vi "log appender.vi"(8 "error in (no error)":errorcluster caption="에러 입력(에러 없음)", 11 "GUI Log Class 입력":refnum<class "GUI Log Class.lvclass">) -> (0 "error out":errorcluster caption="에러 출력")   [LabVIEW 2020, in "GUI Log Class.lvclass"]
uses:
  GUI Log Class.lvclass
  GUI Log Class.lvclass/GUI Log Class.ctl
  Controls/line limit fgv enum.ctl
  Accessors/Read log ref.vi
  Accessors/Read appender queue.vi
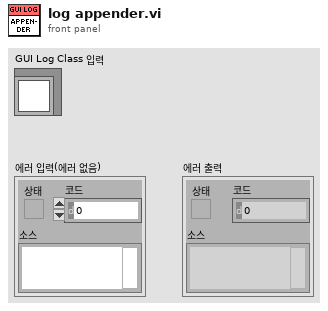
[diagram p1: front panel]
types:
  T1 = typedef "GUI Log Class.lvclass/line limit fgv enum.ctl" = enum16{"Read", "Write"}
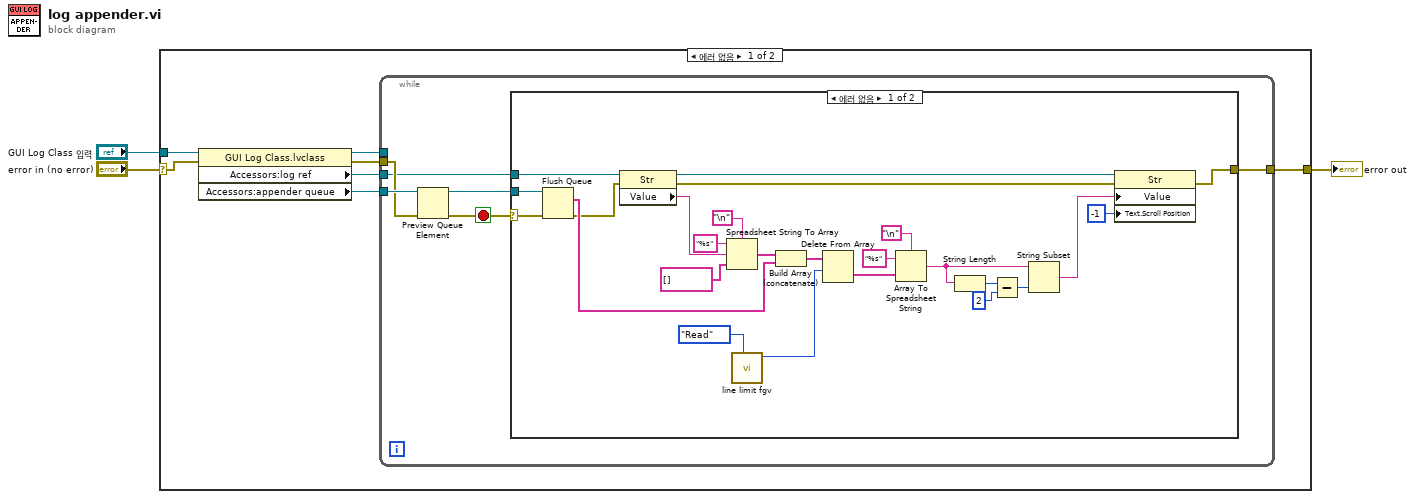
[diagram p0: block diagram]
diagram:
  n1 = case shown="에러 없음" "error in (no error)" {
    selector: "error in (no error)" -> [w10 w43]
    tunnel: [w5 w43] -> w2
    tunnel: "GUI Log Class 입력" -> [w9 _]
    frame No Error {
      n2 = property class="GUI Log Class.lvclass"(reference=w9, error in=w10) -> (reference out=w8:refnum<class "GUI Log Class.lvclass">, error out=w7:errorcluster, "Accessors:log ref"=w4:refnum<vi>, "Accessors:appender queue"=w6:refnum<queue>)
      n3 = while {
        tunnel: w8 -> [_]
        tunnel: w7 -> [w15]
        tunnel: w6 -> [w16]
        tunnel: [w14] -> w5
        tunnel: w4 -> [w11]
        stop <- w12 stop-if-true
        n4 = Preview Queue Element(queue=w16, error in (no error)=w15) -> (queue out=w13:refnum<queue>, error out=w12:errorcluster)  [unwired: 1 in, 2 out]
        n5 = case shown="에러 없음" w12 {
          selector: w12 -> [w40 w42]
          tunnel: [w21 w42] -> w14
          tunnel: w13 -> [w41 _]
          tunnel: w11 -> [w20 _]
          frame No Error {
            n6 = Flush Queue(queue=w41, error in (no error)=w40) -> (remaining elements=w25:string[], error out=w19:errorcluster)  [unwired: 1 out]
            n7 = property class="Str"(reference=w20, error in=w19) -> (reference out=w36:refnum<vi>, error out=w24:errorcluster, "Value"=w31:string)
            n8 = Spreadsheet String To Array(delimiter (Tab)="\n" ("구분 문자 (탭)"), format string="%s" ("포맷 문자열"), spreadsheet string=w31, array type (2D Dbl)=string[] []) -> (array=w27:string[])
            n9 = call "line limit fgv.vi"("function"=line_limit_fgv_enum."Read") -> ("line limit out"=w17:i32)  [unwired: 9 in, 1 out]
            n10 = Build Array (concatenate)(w27, w25) -> (w26:string[])
            n11 = Delete From Array(array=w26, length=w17) -> (deleted portion=w23:string[])  [unwired: 1 in, 1 out]
            n12 = Array To Spreadsheet String(delimiter (Tab)="\n", array=w23, 3:"%s" ("포맷 문자열")) -> (spreadsheet string=w35:string)
            n13 = String Length(string=w35) -> (length=w34:i32)
            n14 = Subtract(x=w34, y=2) -> (x-y=w33:i32)
            n15 = String Subset(string=w35, length (rest)=w33) -> (substring=w22:string)  [unwired: 1 in]
            n16 = property class="Str"(reference=w36, error in=w24, "Value"=w22, "Text.Scroll Position"=-1 ("텍스트.스크롤 위치")) -> (error out=w21:errorcluster)  [unwired: 1 out]
          }
          frame Error {
          }
        }
      }
    }
    frame Error {
    }
  }
  "error out" <- w2
